vi "Butterfly_PullDown RC.vi"(0 "Semiconductor Module Context":T1, 3 "RFPins":string[](array[string]), 5 "error in (no error)":errorcluster, 9 "Start_v":dbl=10.0 format="%#_13g", 11 "Stop_v":dbl=41.0 format="%#_13g") -> (14 "Semiconductor Module Context Out":T1, 19 "error out":errorcluster)   [LabVIEW 2013]
uses:
  <vilib>/NI_TestStand_SemiconductorModule/NI_TestStand_Semiconductor_Module.lvlibp/PinMap/General/SemiconductorModuleContext.ctl
  <instrlib>/niDCPower/nidcpower.llb/niDCPower Wait For Event - Event.ctl
  <vilib>/NI_TestStand_SemiconductorModule/NI_TestStand_Semiconductor_Module.lvlibp/PinMap/DC Power/PinsToNIDCPowerSessions.vi
  <vilib>/NI_TestStand_SemiconductorModule/NI_TestStand_Semiconductor_Module.lvlibp/PinMap/General/Publish/PublishDataDoubleFunctionalTest.vi
  <vilib>/NI_TestStand_SemiconductorModule/NI_TestStand_Semiconductor_Module.lvlibp
panel:
  out "BF values":dbl[](array[numeric])
  out "Full Array":dbl[][][](array[numeric])
  out "BF Names":string[](array[string])
  in  "current level":dbl=0.01 format="%_6p"
  out "R Array":dbl[](array[numeric])
  out "BFSamples":i32
  in  "Step_v":dbl=1.0
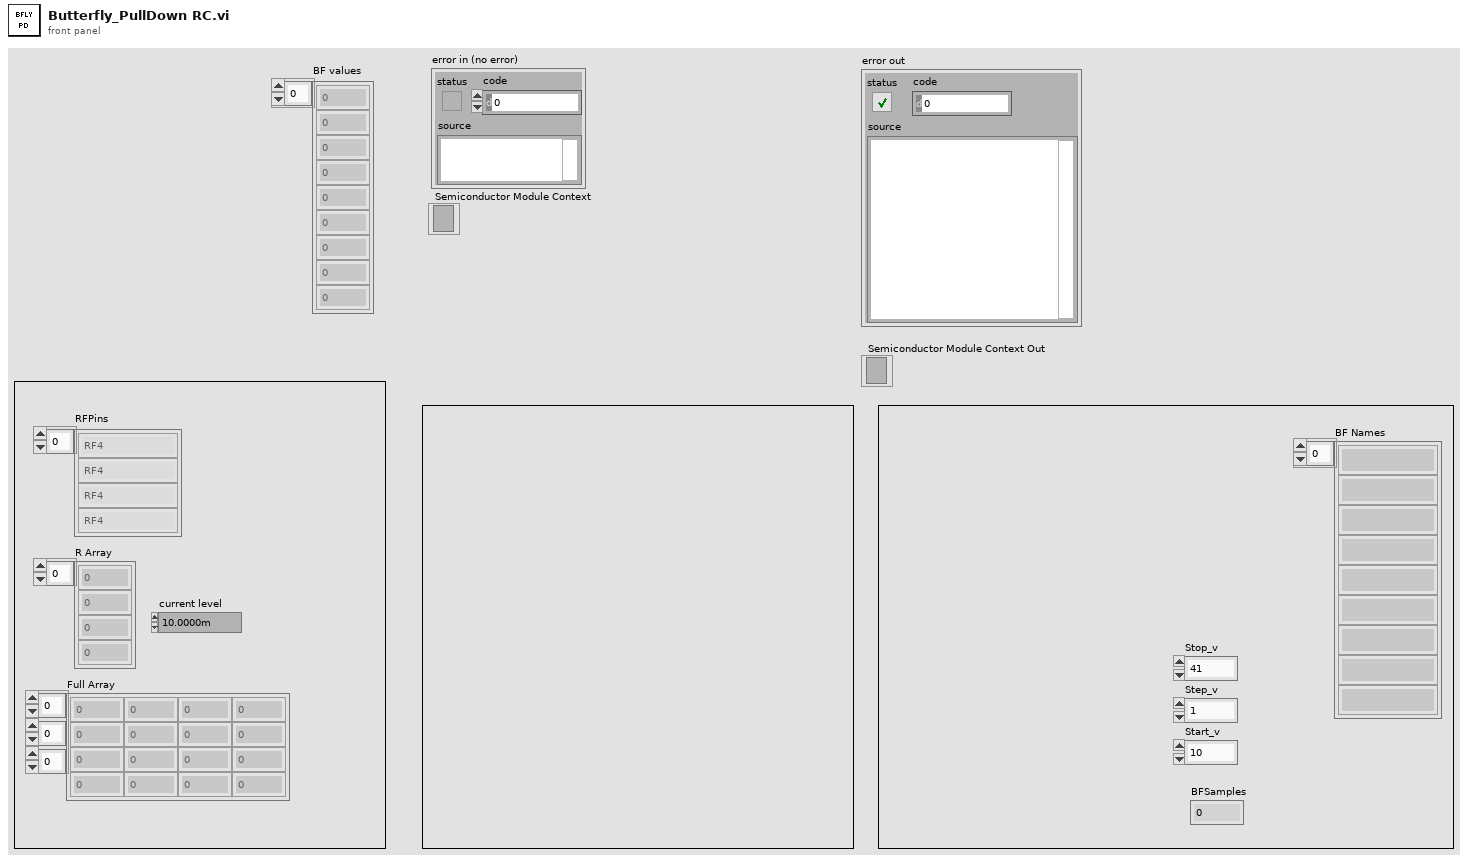
[diagram p1: front panel]
types:
  T1 = typedef "NI_TestStand_Semiconductor_Module.lvlibp/SemiconductorModuleContext.ctl" = refnum<k7>
  T2 = typedef "niDCPower Wait For Event - Event.ctl" = i32
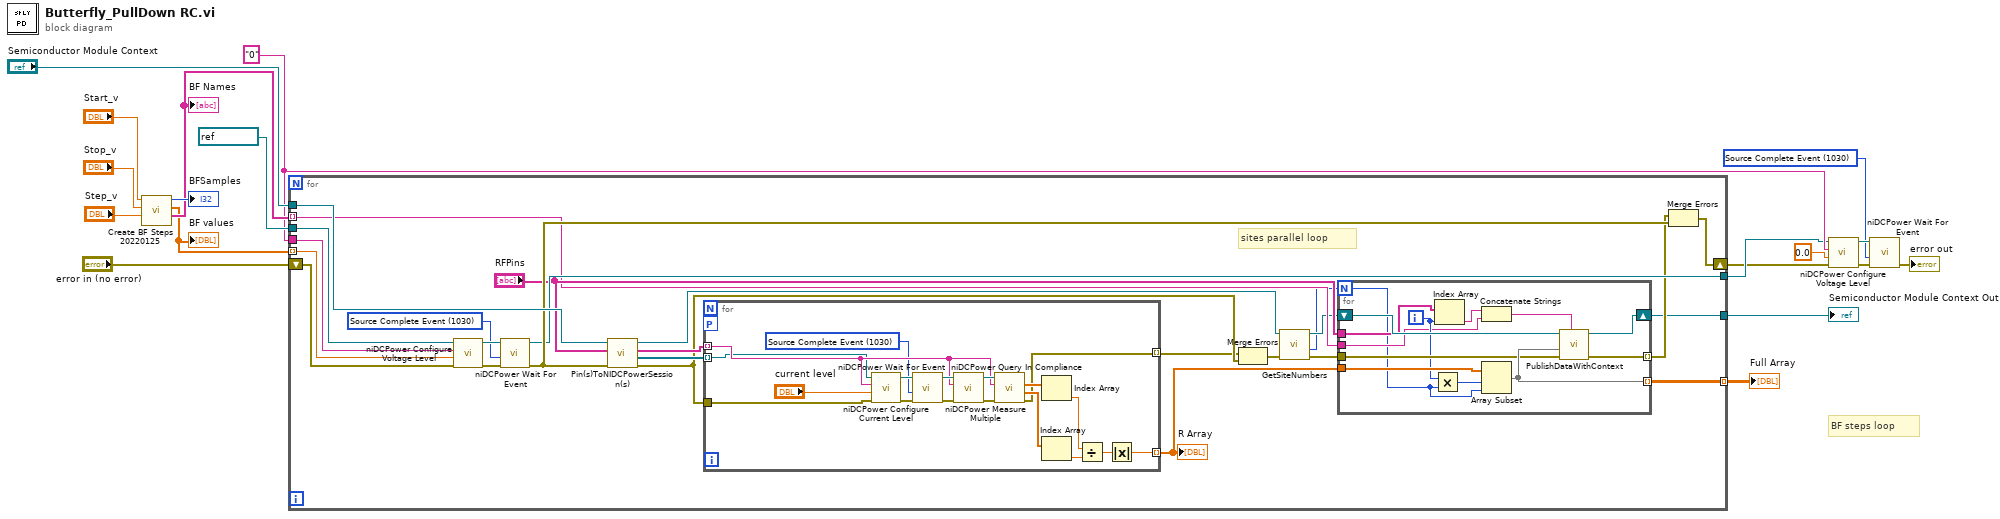
[diagram p0: block diagram]
diagram:
  w5 = T2 1030 items=["Source Complete Event"=1030, "Measure Complete Event"=1031, "Sequence Iteration Complete Event"=1032, "Sequence Engine Done Event"=1033, "Pulse Complete Event"=1051, "Ready For Pulse Trigger Event"=1052] ("event")
  w10 = "0" ("channel name")
  # "BF steps loop"
  n1 = call "Create BF Steps 20220125.vi"("Step_v"="Step_v", "Stop_v"="Stop_v", "Start_v"="Start_v") -> ("BF Names"=w14:string[], "BF values"=w4:dbl[], "BFSamples"=→"BFSamples":i32)  [unwired: 6 in]
  "BF Names" <- w14
  "BF values" <- w4
  n2 = for {
    shift-right: [w21] -> w2
    shift-left: "error in (no error)" -> [w41]
    tunnel: "Semiconductor Module Context" -> [w45]
    tunnel: w14 -> [w27] mode=indexing
    tunnel: w4 -> [w39] mode=indexing
    tunnel: w10 -> [w38]
    tunnel: refnum<k15> "4139_1" ("instrument handle") -> [w37]
    tunnel: [w36] -> w9
    tunnel: [w29] -> w3 mode=indexing
    tunnel: [w20] -> w1
    w43 = T2 1030 items=["Source Complete Event"=1030, "Measure Complete Event"=1031, "Sequence Iteration Complete Event"=1032, "Sequence Engine Done Event"=1033, "Pulse Complete Event"=1051, "Ready For Pulse Trigger Event"=1052] ("event")
    # "sites parallel loop"
    n3 = call <instrlib>:"niDCPower Configure Voltage Level.vi"("error in (no error)"=w41, "voltage level"=w39, "channel name"=w38, "instrument handle"=w37) -> ("error out"=w42:errorcluster, "instrument handle out"=w44:refnum<k15>)  [unwired: 6 in]
    n4 = call <instrlib>:"niDCPower Wait For Event.vi"("error in (no error)"=w42, "event"=w43, "instrument handle"=w44) -> ("error out"=w40:errorcluster, "instrument handle out"=w36:refnum<k15>)  [unwired: 7 in]
    n5 = call-poly <vilib>:"Pin(s)ToNIDCPowerSession(s).vi"("error in (no error)"=w40, "Pins"="RFPins", "Semiconductor Module Context"=w45) -> ("error out"=w33:errorcluster, "Instrument Sessions"=w34:refnum<k15>[], "Channel Lists"=w35:string[], "Semiconductor Module Context Out"=w26:T1)  [unwired: 4 in, 1 out]
    n6 = for {
      tunnel: w35 -> [w63] mode=indexing
      tunnel: w34 -> [w59] mode=indexing
      tunnel: w33 -> [w60]
      tunnel: [w64] -> w31 mode=indexing
      tunnel: [w61] -> w32 mode=indexing
      workers-P: _ -> [_]
      w62 = T2 1030 items=["Source Complete Event"=1030, "Measure Complete Event"=1031, "Sequence Iteration Complete Event"=1032, "Sequence Engine Done Event"=1033, "Pulse Complete Event"=1051, "Ready For Pulse Trigger Event"=1052] ("event")
      n7 = call <instrlib>:"niDCPower Configure Current Level.vi"("error in (no error)"=w60, "current level"="current level", "channel name"=w63, "instrument handle"=w59) -> ("error out"=w72:errorcluster, "instrument handle out"=w71:refnum<k15>)  [unwired: 6 in]
      n8 = call <instrlib>:"niDCPower Wait For Event.vi"("error in (no error)"=w72, "event"=w62, "instrument handle"=w71) -> ("error out"=w76:errorcluster, "instrument handle out"=w75:refnum<k15>)  [unwired: 7 in]
      n9 = call <instrlib>:"niDCPower Query In Compliance.vi"("error in (no error)"=w76, "channel name"=w63, "instrument handle"=w75) -> ("error out"=w73:errorcluster, "instrument handle out"=w74:refnum<k15>)  [unwired: 6 in, 1 out]
      n10 = call <instrlib>:"niDCPower Measure Multiple.vi"("error in (no error)"=w73, "channel name"=w63, "instrument handle"=w74) -> ("error out"=w61:errorcluster, "current measurements"=w65:dbl[], "voltage measurements"=w66:dbl[])  [unwired: 5 in, 1 out]
      n11 = Index Array(array=w66) -> (element=w68:dbl)  [unwired: 1 in]
      n12 = Index Array(array=w65) -> (element=w67:dbl)  [unwired: 1 in]
      n13 = Divide(x=w68, y=w67) -> (x/y=w69:dbl)
      n14 = Absolute Value(x=w69) -> (abs(x)=w64:dbl)
    }
    "R Array" <- w31
    n15 = Merge Errors(w32, w33) -> (w24:errorcluster)
    n16 = call <vilib>:"GetSiteNumbers.vi"("error in (no error)"=w24, "Semiconductor Module Context"=w26) -> ("error out"=w23:errorcluster, "Number Of Sites"=w22:i32, "Semiconductor Module Context Out"=w25:T1)  [unwired: 6 in, 1 out]
    n17 = for {
      N: w22 -> [w46]
      tunnel: w31 -> [w58]
      tunnel: [w55] -> w29 mode=indexing
      tunnel: w23 -> [w54]
      tunnel: [w52] -> w30 mode=indexing
      shift-right: [w53] -> w20
      shift-left: w25 -> [w56]
      tunnel: "RFPins" -> [w50]
      tunnel: w27 -> [w47]
      i -> [w49]
      n18 = Multiply(x=w49, y=w46) -> (x*y=w57:i32)
      n19 = Index Array(array=w50, index=w49) -> (element=w48:string)
      n20 = Concatenate Strings(w48, w47) -> (w51:string)
      n21 = Array Subset(array=w58, index=w57, length=w46) -> (w55:dbl[])
      n22 = call-poly <vilib>:"PublishDataWithContext.vi"("Published Data Id"=w51, "error in (no error)"=w54, "Data In"=w55, "Semiconductor Module Context"=w56) -> ("error out"=w52:errorcluster, "Semiconductor Module Context Out"=w53:T1)  [unwired: 6 in]
    }
    n23 = Merge Errors(w30, w40) -> (w21:errorcluster)
  }
  "Semiconductor Module Context Out" <- w1
  "Full Array" <- w3
  n24 = call <instrlib>:"niDCPower Configure Voltage Level.vi"("error in (no error)"=w2, "voltage level"=0.0, "channel name"=w10, "instrument handle"=w9) -> ("error out"=w8:errorcluster, "instrument handle out"=w6:refnum<k15>)  [unwired: 6 in]
  n25 = call <instrlib>:"niDCPower Wait For Event.vi"("error in (no error)"=w8, "event"=w5, "instrument handle"=w6) -> ("error out"=→"error out":errorcluster)  [unwired: 7 in, 1 out]
